vi "Write Input Registers.vi"(8 "error in (no error)":errorcluster, 9 "register values":u16[](array[numeric]), 10 "starting address":u16, 11 "device data model in":refnum<class "Device Data Model.lvclass">) -> (0 "error out":errorcluster, 3 "device data model out":refnum<class "Device Data Model.lvclass">)   [LabVIEW 2018, in "SubVIs.lvlib" / "Device Data Model.lvclass"]
doc: "Writes the values of multiple input register values in series, starting at address M."
uses:
  Device Data Model.lvclass
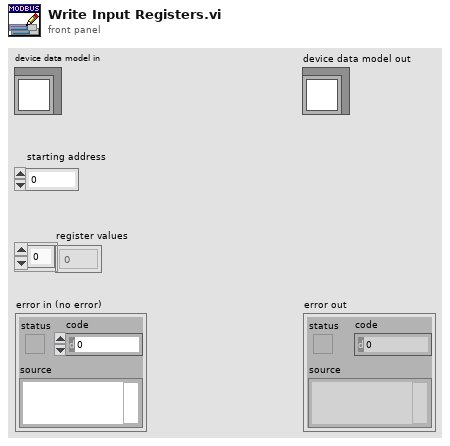
[diagram p1: front panel]
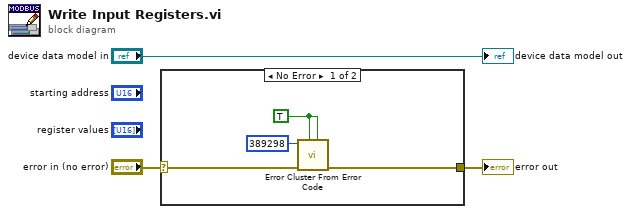
[diagram p0: block diagram]
diagram:
  n1 = case shown="No Error" "error in (no error)" {
    selector: "error in (no error)" -> [w6 w8]
    tunnel: [w7 w8] -> w1
    frame No Error {
      w4 = TRUE ("show call chain? (False)")
      n2 = call "Error Cluster From Error Code.vi"("is warning? (False)"=w4, "show call chain? (False)"=w4, "error in (no error)"=w6, "error code (0)"=389298) -> ("error out"=w7:errorcluster)  [unwired: 5 in]
    }
    frame Error {
    }
  }
  "error out" <- w1
  "device data model out" <- "device data model in"
